vi "_PC_RTFunc_ReadTurboPumpStatus.vi"(8 "error in (no error)":errorcluster) -> (0 "error out":errorcluster, 1 "Time Stamp":timestamp, 2 "TurboStatus_string":string, 4 "valid":bool)   [LabVIEW 2018]
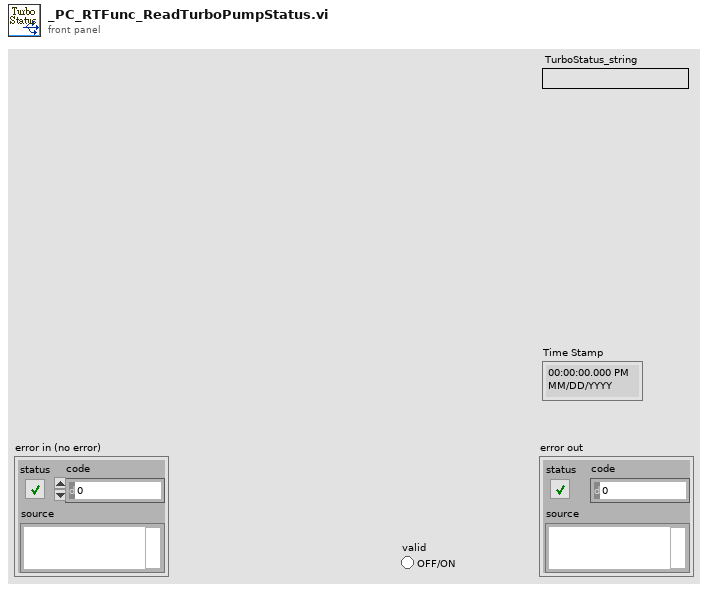
[diagram p1: front panel]
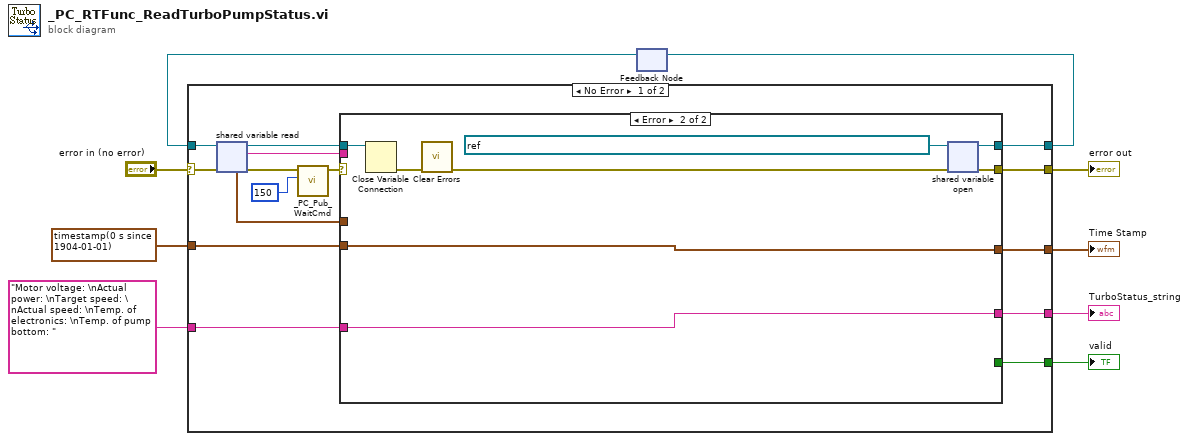
[diagram p0: block diagram]
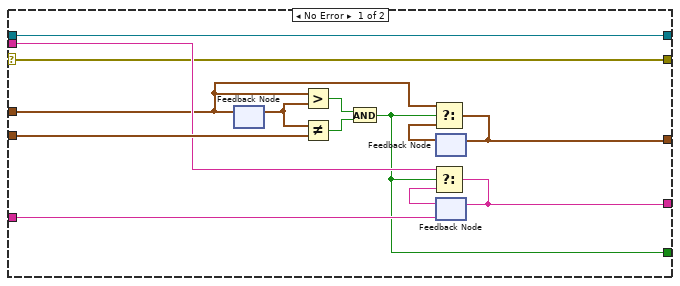
[diagram p2: hidden frame]
diagram:
  n1 = feedback #1() -> (w7:refnum<k21>)  [unwired: 1 in]
  n2 = case shown="No Error" "error in (no error)" {
    selector: "error in (no error)" -> [w24 w47]
    tunnel: [w21 w50] -> w8
    tunnel: w7 -> [w20 w50]
    tunnel: [w19 w48] -> w3
    tunnel: [w17 w49] -> w5
    tunnel: timestamp(0 s since 1904-01-01) -> [w16 w49]
    tunnel: "Motor voltage: \nActual power: \nTarget speed: \nActual speed: \nTemp. of electronics: \nTemp. of pump bottom: " ("format string") -> [w15 w48]
    tunnel: [w14 w47] -> w2
    tunnel: [w10 _] -> w1
    frame No Error {
      n3 = shared-variable-read(w20, w24) -> (w22:refnum<k21>, w13:errorcluster, w23:string, w18:timestamp)
      n4 = call "_PC_Pub_WaitCmd.vi"("milliseconds to wait"=u32 150, "error in (no error)"=w13) -> ("error out"=w12:errorcluster)  [unwired: 9 in]
      n5 = case shown="Error" w12 {
        selector: w12 -> [w27 _]
        tunnel: w23 -> [w34 _]
        tunnel: w22 -> [w38 w46]
        tunnel: [w38 w42] -> w21
        tunnel: [w29 w40] -> w19
        tunnel: w18 -> [w26 _]
        tunnel: [w28 w41] -> w17
        tunnel: w16 -> [w37 w41]
        tunnel: w15 -> [w32 w40]
        tunnel: [w27 w39] -> w14
        tunnel: [w25 _] -> w10
        frame No Error {
          n6 = feedback #2() -> (w36:timestamp)  [unwired: 1 in]
          n7 = feedback-in #2(w26) -> ()
          n8 = Greater?(x=w26, y=w36) -> (0:w31:bool)
          n9 = Not Equal?(x=w36, y=w37) -> (x != y?=w30:bool)
          n10 = And(x=w31, y=w30) -> (x .and. y?=w25:bool)
          n11 = feedback #3() -> (w35:timestamp)  [unwired: 1 in]
          n12 = Select(t=w26, s=w25, f=w35) -> (s? t:f=w28:timestamp)
          n13 = feedback-in #3(w28) -> ()
          n14 = feedback #4(w32) -> (w33:string)
          n15 = Select(t=w34, s=w25, f=w33) -> (s? t:f=w29:string)
          n16 = feedback-in #4(w29) -> ()
        }
        frame Error {
          n17 = Close Variable Connection(11:w46) -> (0:w45:errorcluster)  [unwired: 1 in]
          n18 = call <vilib>:"Clear Errors.vi"("error in (no error)"=w45) -> ("error out"=w43:errorcluster)  [unwired: 5 in, 1 out]
          n19 = shared-variable-open(refnum<k21> "ni.var.psp://NI-sbRIO/_RT_CtrlLoop_TurboPump_Variables/TurboStatus_string" ("shared variable refnum in"), w43) -> (w42:refnum<k21>, w39:errorcluster)
        }
      }
    }
    frame Error {
    }
  }
  "error out" <- w2
  "Time Stamp" <- w5
  "TurboStatus_string" <- w3
  "valid" <- w1
  n20 = feedback-in #1(w8) -> ()
